vi "Init Events.vi"(8 "error in (no error)":errorcluster, 11 "Basic WebSocket Manager in":refnum<class "Basic WebSocket Manager.lvclass">) -> (0 "error out":errorcluster, 3 "Basic WebSocket Manager out":refnum<class "Basic WebSocket Manager.lvclass">)   [LabVIEW 2020, in "HTTP Server.lvlib" / "Basic WebSocket Manager.lvclass"]
uses:
  Basic WebSocket Manager.lvclass
  Create Client Data.ctl
  lv-http-util/HTTP Utils/Request/Request.lvclass
  lv-promises/Promises/Promise/Promise.lvclass
  Events.ctl
  Basic WebSocket Manager.lvclass/Basic WebSocket Manager.ctl
  WebSocket Client/WebSocket Client.lvclass
  Client Ready Data.ctl
  Client Closed Data.ctl
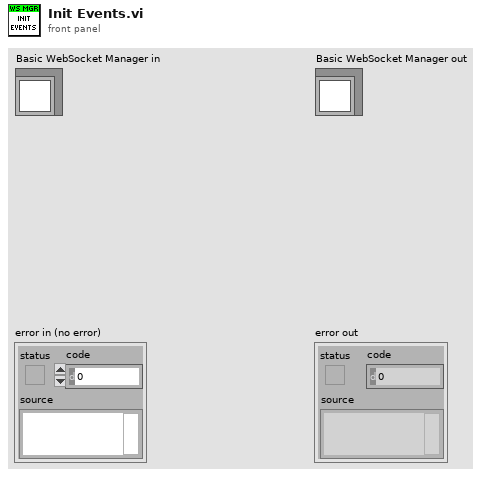
[diagram p1: front panel]
types:
  T1 = typedef "HTTP Server.lvlib/Basic WebSocket Manager.lvclass/Client Closed Data.ctl" = cluster{"Client":refnum<class "WebSocket Client.lvclass">}
  T2 = typedef "HTTP Server.lvlib/Basic WebSocket Manager.lvclass/Client Ready Data.ctl" = cluster{"Client":refnum<class "WebSocket Client.lvclass">}
  T3 = typedef "HTTP Server.lvlib/Basic WebSocket Manager.lvclass/Events.ctl" = cluster{"Create Client":refnum<user-event>, "Client Ready":refnum<user-event>, "Client Closed":refnum<user-event>}
  T4 = typedef "HTTP Server.lvlib/Basic WebSocket Manager.lvclass/Create Client Data.ctl" = cluster{"Request":refnum<class "Request.lvclass">, "TCP":refnum<k5>, "Promise":refnum<class "Promise.lvclass">}
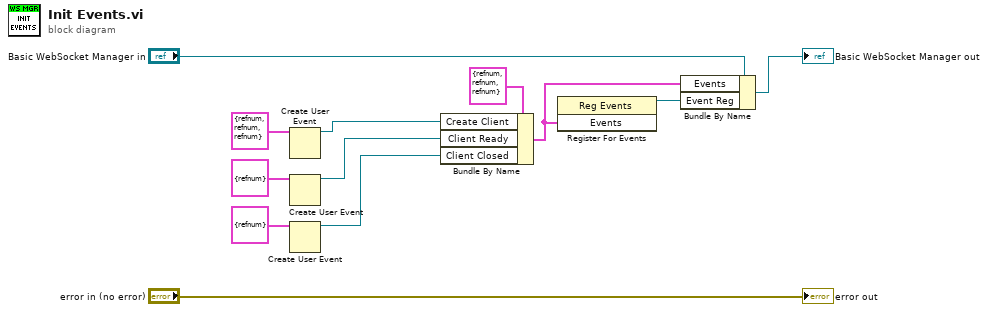
[diagram p0: block diagram]
diagram:
  n1 = Create User Event(user event datatype=T4 {"Request"=refnum, "TCP"=refnum, "Promise"=refnum} ("Create Client Data")) -> (user event=w8:refnum<user-event>)  [unwired: 1 in, 1 out]
  n2 = Create User Event(user event datatype=T2 {"Client"=refnum} ("Client Ready Data")) -> (user event=w2:refnum<user-event>)  [unwired: 1 in, 1 out]
  n3 = Create User Event(user event datatype=T1 {"Client"=refnum} ("Client Closed Data")) -> (user event=w1:refnum<user-event>)  [unwired: 1 in, 1 out]
  n4 = Bundle By Name(cluster=T3 {"Create Client"=refnum, "Client Ready"=refnum, "Client Closed"=refnum} ("Events"), "Create Client"=w8, "Client Ready"=w2, "Client Closed"=w1) -> (w5:T3)
  n5 = register-events(w5) -> (reference out=w6:refnum<event-registration>)  [unwired: 2 in, 1 out]
  n6 = Bundle By Name(cluster="Basic WebSocket Manager in", "Events"=w5, "Event Reg"=w6) -> (→"Basic WebSocket Manager out":refnum<class "Basic WebSocket Manager.lvclass">)
  "error out" <- "error in (no error)"
